vi "单元格是否在范围内.vi"(8 "error in (no error)":errorcluster caption="错误输入（无错误）", 10 "行列范围":cluster{"起始行列":T1, "结束行列":T1}, 11 "单元格位置":T1 caption="表格位置") -> (0 "error out":errorcluster caption="错误输出", 2 "是否在范围":bool, 3 "单元格位置输出":T1 caption="表格位置")   [LabVIEW 2014, in "表格.lvlib"]
uses:
  <vilib>/Utility/miscctls.llb/LVRowAndColumnTypeDef.ctl
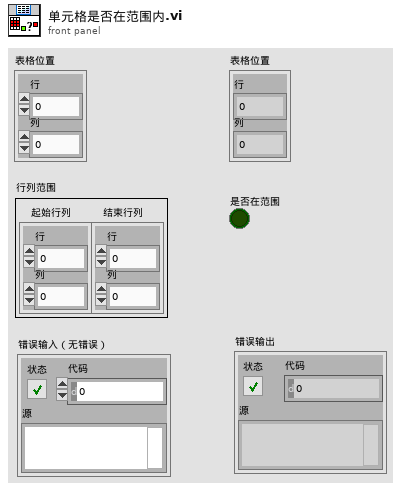
[diagram p1: front panel]
types:
  T1 = typedef "LVRowAndColumnTypeDef.ctl" = cluster{"Row":i32, "Column":i32}
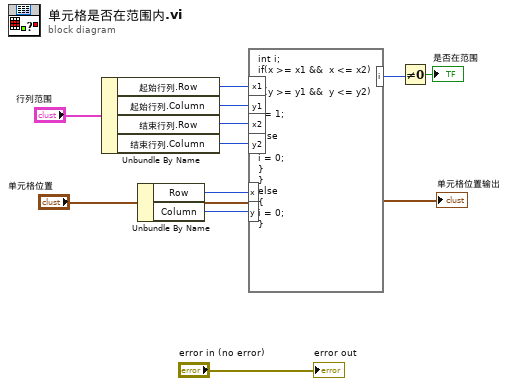
[diagram p0: block diagram]
diagram:
  n1 = Unbundle By Name("行列范围") -> ("起始行列.Row"=w6:i32, "起始行列.Column"=w7:i32, "结束行列.Row"=w8:i32, "结束行列.Column"=w9:i32)
  n2 = Unbundle By Name("单元格位置") -> ("Row"=w5:i32, "Column"=w4:i32)
  n3 = formula code="int i;\nif(x >= x1 &&  x <= x2)\n{\nif(y >= y1 &&  y <= y2)\n{\ni = 1;\n}\nelse\n{\ni = 0;\n}\n}\nelse\n{\ni = 0;\n}"("x1"=w6, "y1"=w7, "x2"=w8, "y2"=w9, "x"=w5, "y"=w4) -> ("i"=w3:i32)
  n4 = Not Equal To 0?(x=w3) -> (x != 0?=→"是否在范围":bool)
  "单元格位置输出" <- "单元格位置"
  "error out" <- "error in (no error)"
